vi "KeyenceCVX.Main.ScanAck.Init.vi"(4 "get image":bool, 6 "Retries (-1: Default)":i32=-1, 7 "TriggerNo":T4 items=["1"=1, "2"=2, "3"=3, "4"=4, "ALL"=5], 8 "error in":errorcluster, 9 "ImgPath":path, 11 "Data":T1 {"Status"."TriggerNo" items=["1"=1, "2"=2, "3"=3, "4"=4, "ALL"=5]}) -> (0 "error out":errorcluster, 2 "started":bool, 3 "Data out":T1 {"Status"."TriggerNo" items=["1"=1, "2"=2, "3"=3, "4"=4, "ALL"=5]})   [LabVIEW 2016]
uses:
  KeyenceCVX.Data.ctl
  KeyenceCVX.Data.Status.ctl
  KeyenceCVX.Data.Status.State.ctl
  private/controls/TriggerNo.ctl
  KeyenceCVX.Data.Sets.ctl
  KeyenceCVX.CodeDetails.ctl
  Keyence/LowLevel/Keyence.Global.vi
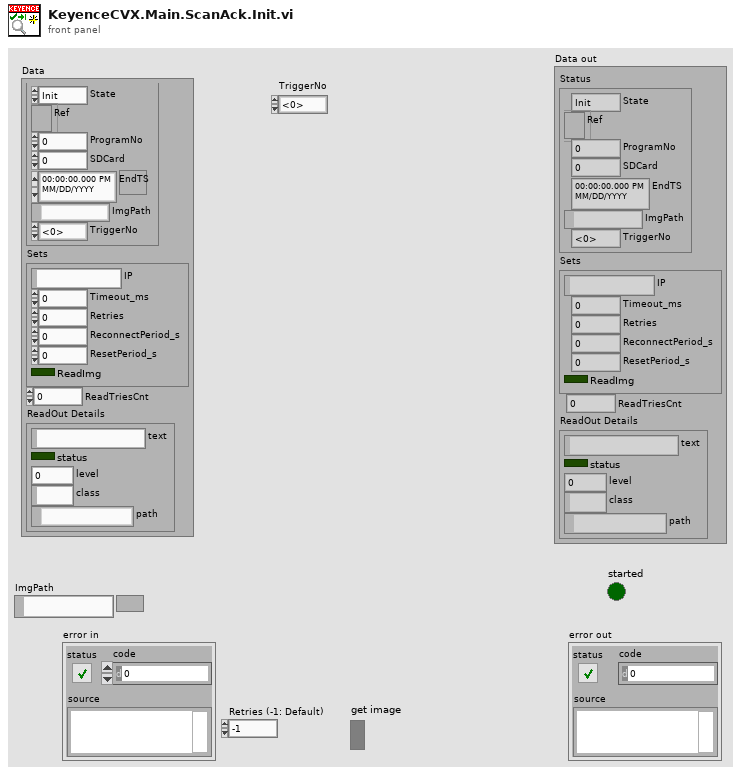
[diagram p1: front panel]
types:
  T1 = typedef "KeyenceCVX.Data.ctl" = cluster{"Status":T2, "Sets":T5, "ReadTriesCnt":u8, "ReadOut Details":T6}
  T2 = typedef "KeyenceCVX.Data.Status.ctl" = cluster{"State":T3, "Ref":refnum<k5>, "ProgramNo":u16, "SDCard":u8, "EndTS":timestamp, "ImgPath":path, "TriggerNo":T4}
  T3 = typedef "KeyenceCVX.Data.Status.State.ctl" = enum16{"Init", "Idle", "Scan", "Reset", "ScanAck"}
  T4 = typedef "TriggerNo.ctl" = u8
  T5 = typedef "KeyenceCVX.Data.Sets.ctl" = cluster{"IP":string, "Timeout_ms":i32, "Retries":i32, "ReconnectPeriod_s":i32, "ResetPeriod_s":i32, "ReadImg":bool}
  T6 = typedef "KeyenceCVX.CodeDetails.ctl" = cluster{"text":string, "status":bool, "level":u8, "class":string, "path":path}
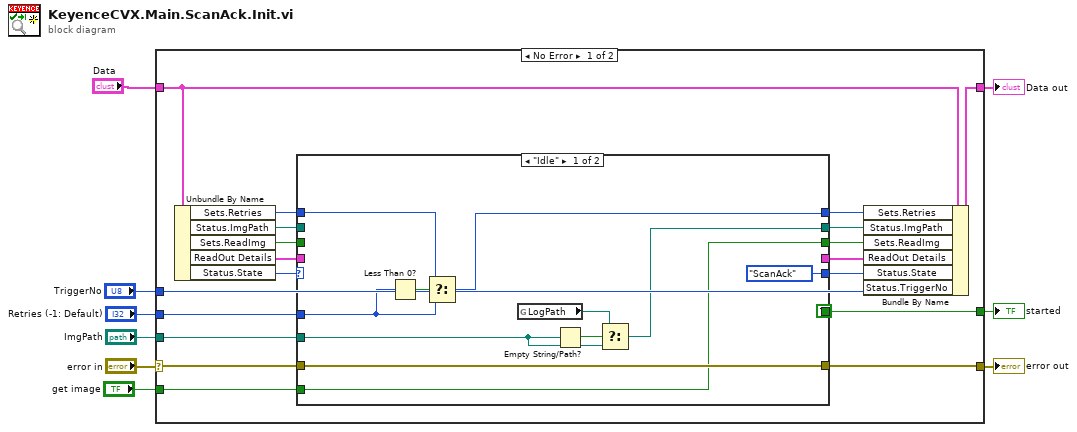
[diagram p0: block diagram]
diagram:
  n1 = case shown="No Error" "error in" {
    selector: "error in" -> [w24 w48]
    tunnel: [w26 w48] -> w8
    tunnel: "Data" -> [w27 w47]
    tunnel: [w28 w47] -> w1
    tunnel: [w20 _] -> w7
    tunnel: "ImgPath" -> [w19 _]
    tunnel: "Retries (-1: Default)" -> [w16 _]
    tunnel: "get image" -> [w11 _]
    tunnel: "TriggerNo" -> [w10 _]
    frame No Error {
      n2 = Unbundle By Name(w27) -> ("Sets.Retries"=w14:i32, "Status.ImgPath"=w17:path, "Sets.ReadImg"=w13:bool, "ReadOut Details"=w22:T6, "Status.State"=w25:T3)
      n3 = case shown="\"Idle\"" w25 {
        selector: w25 -> [_ w46]
        tunnel: w24 -> [w40 w44]
        tunnel: [w40 w44] -> w26
        tunnel: [KeyenceCVX.Data.Status.State."ScanAck" ("State") w46] -> w23
        tunnel: [_ w45] -> w21
        tunnel: w22 -> [_ w45]
        tunnel: [TRUE _] -> w20
        tunnel: w19 -> [w36 _]
        tunnel: [w35 w43] -> w18
        tunnel: w17 -> [_ w43]
        tunnel: w16 -> [w31 _]
        tunnel: [w32 w42] -> w15
        tunnel: w14 -> [w33 w42]
        tunnel: w13 -> [_ w41]
        tunnel: [w30 w41] -> w12
        tunnel: w11 -> [w30 _]
        frame "Idle" {
          n4 = Less Than 0?(x=w31) -> (x < 0?=w34:bool)
          n5 = Select(t=w33, s=w34, f=w31) -> (s? t:f=w32:i32)
          n6 = global read "Keyence.Global.vi" "LogPath"() -> (w37:path)
          n7 = Empty String/Path?(string/path=w36) -> (empty?=w38:bool)
          n8 = Select(t=w37, s=w38, f=w36) -> (s? t:f=w35:path)
        }
        frame Default {
        }
      }
      n9 = Bundle By Name(cluster=w27, "Sets.Retries"=w15, "Status.ImgPath"=w18, "Sets.ReadImg"=w12, "ReadOut Details"=w21, "Status.State"=w23, "Status.TriggerNo"=w10) -> (w28:T1)
    }
    frame Error {
    }
  }
  "error out" <- w8
  "started" <- w7
  "Data out" <- w1
